vi "Init Connection.vi"(8 "error in (no error)":errorcluster, 10 "ApiKey":string) -> (0 "error out":errorcluster, 3 "client handle out":T1)   [LabVIEW 2019]
uses:
  <vilib>/httpClient/ClientHandle.ctl
  <vilib>/httpClient/LabVIEWHTTPClient.lvlib
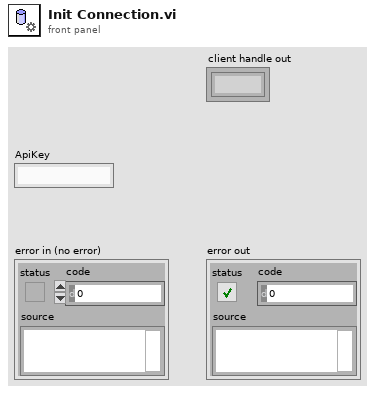
[diagram p1: front panel]
types:
  T1 = typedef "LabVIEWHTTPClient.lvlib/ClientHandle.ctl" = refnum<k1>
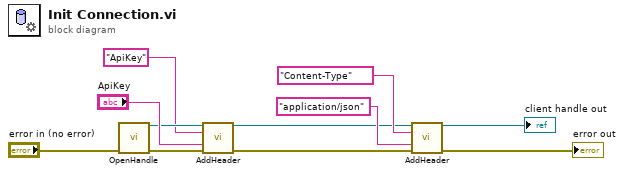
[diagram p0: block diagram]
diagram:
  n1 = call <vilib>:"OpenHandle.vi"("error in (no error)"="error in (no error)") -> ("client handle out"=w3:T1, "error out"=w4:errorcluster)  [unwired: 13 in]
  n2 = call <vilib>:"AddHeader.vi"("client handle"=w3, "header"="ApiKey" ("url"), "value"="ApiKey", "error in (no error)"=w4) -> ("client handle out"=w8:T1, "error out"=w6:errorcluster)  [unwired: 10 in]
  n3 = call <vilib>:"AddHeader.vi"("client handle"=w8, "header"="Content-Type", "value"="application/json", "error in (no error)"=w6) -> ("client handle out"=→"client handle out":T1, "error out"=→"error out":errorcluster)  [unwired: 10 in]
